vi "Help_difinicao_adq.vi"() -> ()   [LabVIEW 2019]
panel:
  in  "stop":bool
  # "OLÁ, SEJA BEM VINDO AO ADQUIRI\nO PROGRAMA FOI CRIADO COM O OBJETIVO DE ADQUIRIR OS DADOS LIDOS PELA \nPLACA DA NATIONAL INSTRUMENTS NA QUAL MONITORA OS VALORES DE PRESSÕES\nDE CHEIO E VAZIO DAS PLACAS DE IMPEDÂNCIA, QUE ESTÃO LOCALIZADOS NA TORRE\nDE DESLOCAMENTOS DE FLUÍDOS\nO PROGRAMA TEM 2 FUNÇÕES PRINCIPAIS, MOSTRAR EM UM GRÁFICO EM TEMPO REAL\nOS VALORES LIDOS PROVENIENTES DA PLACA, QUE TRABALHA COM UM CERTO\nNÚMERO DE AMOSTRAS\nTAMBÉM, O PROGRAMA É CAPAZ DE ESCREVER OS DADOS EM ARQUIVO TXT"
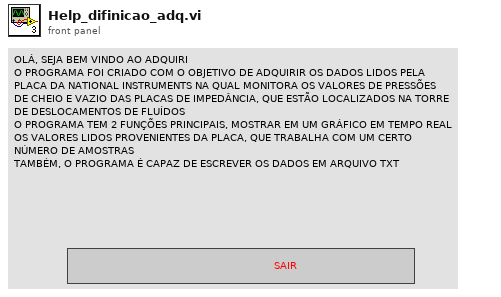
[diagram p1: front panel]
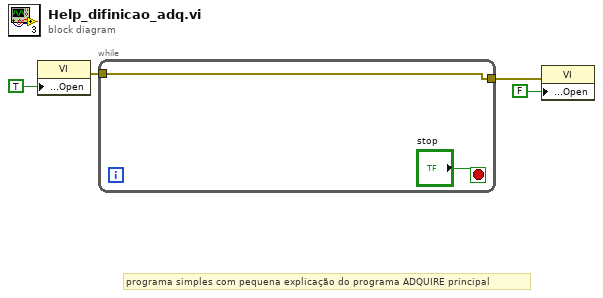
[diagram p0: block diagram]
diagram:
  # "programa simples com pequena explicação do programa ADQUIRE principal"
  n1 = property class="VI"("Front Panel.Open"=TRUE ("Front Panel Window:Open")) -> (error out=w1:errorcluster)  [unwired: 2 in, 1 out]
  n2 = while {
    tunnel: [w5] -> w2
    tunnel: w1 -> [w5]
    stop <- "stop" stop-if-true
  }
  n3 = property class="VI"(error in=w2, "Front Panel.Open"=FALSE ("Front Panel Window:Open")) -> ()  [unwired: 1 in, 2 out]
